vi "GE 5565 Dual Card.vi"() -> ()   [LabVIEW 2016]
uses:
  <vilib>/Utility/RT CPU Load.ctl
  <vilib>/Platform/TimedLoop/XDataNode/timing_clust.ctl
  <vilib>/Platform/TimedLoop/XDataNode/nitl_modes.ctl
  <vilib>/Platform/TimedLoop/XDataNode/wakeup.ctl
  <instrlib>/GE 5565 PIORC/Public/DMA Interrupt/GE5565 DMA Read Interrupt (U8) Cluster.vi
  <vilib>/Platform/TimedLoop/XDataNode/XDataNode.xnode
  <instrlib>/GE 5565 PIORC/GE 5565 PIORC.lvlib
  <vilib>/Platform/TimedLoop/XDataNode/XDNodeRunTimeDep.lvlib
  <vilib>/NI_Real-Time Target Support.lvlib
panel:
  out "w period 2":u32
  out "Times":cluster{u32, u32}
  out "CPU loads":T1[](array[typedef]) {"ISR (%)" format="%#.2f"; "Idle (%)" format="%#.2f"; "Background (%)" format="%#.2f"; "Normal (%)" format="%#.2f"; "Above Normal (%)" format="%#.2f"; "High (%)" format="%#.2g"; "Timed Structures (%)" format="%#.2g"; "Time Critical (%)" format="%#.2g"; "Total (%)" format="%#.2g"}
  in  "mode":enum16{"write", "read"}(ring)
  in  "size":i32=10000
  out "r element":dbl
  in  "r index":i32
  out "r period":u32
  in  "w element":dbl
  in  "w index":i32
  in  "stop":bool
  out "w period":u32
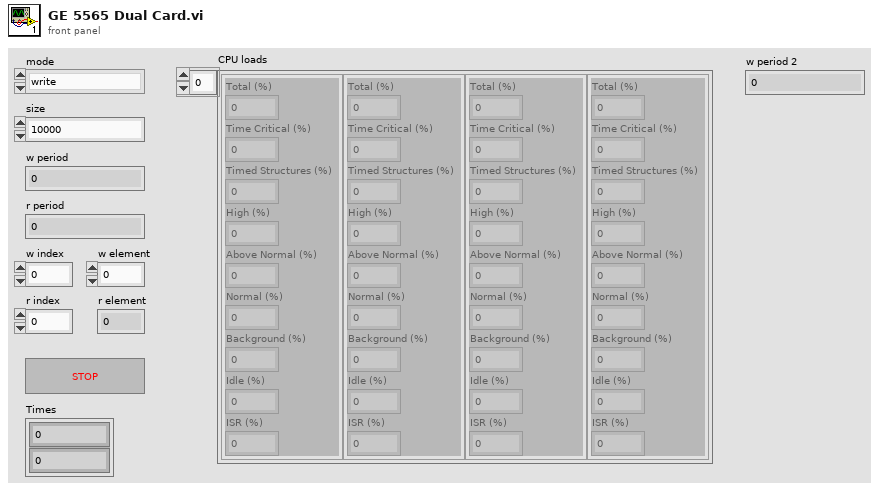
[diagram p1: front panel]
types:
  T1 = typedef "NI_Real-Time Target Support.lvlib/RT CPU Load.ctl" = cluster{"Total (%)":dbl, "Time Critical (%)":dbl, "Timed Structures (%)":dbl, "High (%)":dbl, "Above Normal (%)":dbl, "Normal (%)":dbl, "Background (%)":dbl, "Idle (%)":dbl, "ISR (%)":dbl}
  T2 = typedef "XDNodeRunTimeDep.lvlib/timing_clust.ctl" = cluster{"Expected End [f-1]":u64, "Actual End [f-1]":u64, "Finished Late? [f-1]":bool, "Expected End [i-1]":u64, "Actual End [i-1]":u64, "Finished Late? [i-1]":bool, "Expected Start [i]":u64, "Actual Start [i]":u64, "Expected Start [f]":u64, "Actual Start [f]":u64, "Source Name":string, "Structure Name":string, "Period":i64, "Deadline":i64, "Offset":i64, "Start":i64, "Priority":i32, "Timeout":i32, "Mode":T3, "Wakeup Reason":T4, "Error":errorcluster, "Source Type":string, "Secondary Source Type":string, "Global End Time":u64, "Global Start Time":u64, "Frame Duration":u64, "Iteration Duration":u64, "Assigned CPU":i32, "I/O Scan Engine Mode":u32}
  T3 = typedef "XDNodeRunTimeDep.lvlib/nitl_modes.ctl" = enum32{"No Change", "Process missed periods, maintain original phase", "Discard missed periods, maintain original phase", "Process missed periods, ignore original phase", "Discard missed periods, ignore original phase"}
  T4 = typedef "XDNodeRunTimeDep.lvlib/wakeup.ctl" = enum32{"Normal", "Aborted", "Asynchronous wakeup", "Timing source error", "Timed loop error", "Timeout"}
  T5 = cluster{"VMIC 5565 Resource":refnum<visa-resource-name>, "MEMACC Resource":refnum<visa-resource-name>, "byte count":u32, "mem offset":u32}
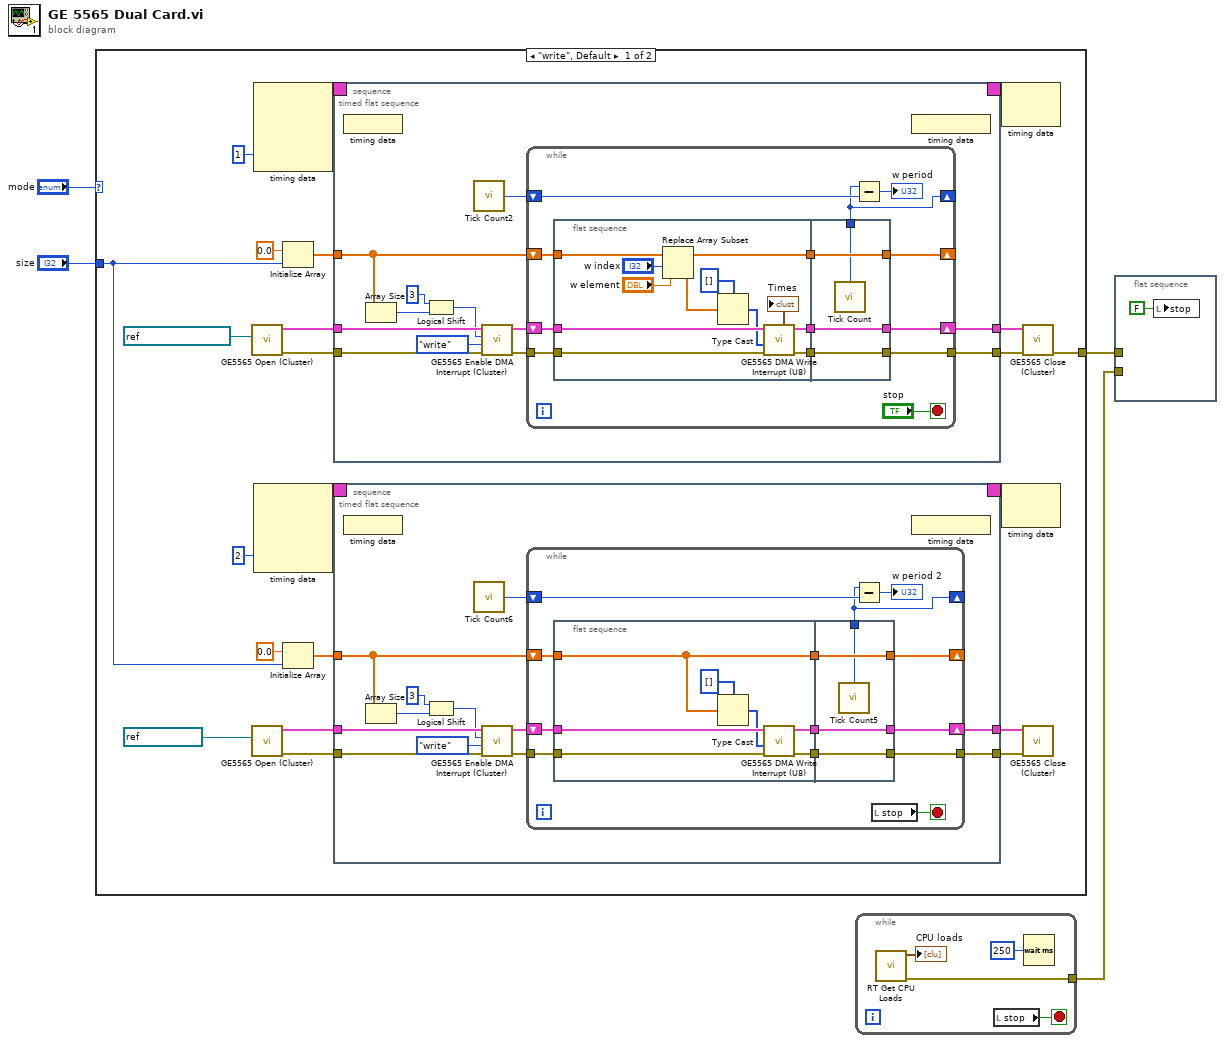
[diagram p0: block diagram]
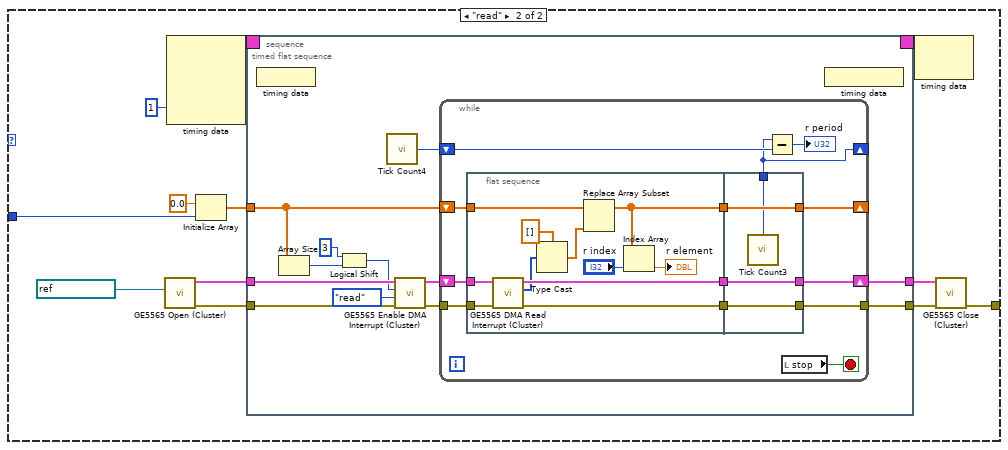
[diagram p2: hidden frame]
diagram:
  n1 = case shown="\"write\", Default" "mode" {
    tunnel: "size" -> [w15 w126]
    tunnel: [w16 w125] -> w2
    frame "write", Default {
      n2 = call <instrlib>:"GE5565 Open (Cluster).vi"("VISA resource name (empty)"=refnum<visa-resource-name> "PXI2::13::INSTR") -> ("error out"=w22:errorcluster, "VMIC-5565"=w23:T5)  [unwired: 5 in]
      n3 = call <instrlib>:"GE5565 Open (Cluster).vi"("VISA resource name (empty)"=refnum<visa-resource-name> "RefMem2") -> ("error out"=w7:errorcluster, "VMIC-5565"=w6:T5)  [unwired: 5 in]
      n4 = node-c288(1 ("Processor")) -> (w26:T2)  [unwired: 3 in]
      n5 = node-c288(2 ("Processor")) -> (w14:T2)  [unwired: 3 in]
      n6 = Initialize Array(0.0 ("element"), w15) -> (w18:dbl[])
      n7 = Initialize Array(0.0 ("element"), w15) -> (w11:dbl[])
      n8 = timed-sequence {
        timing: w26 -> [_]
        timing-out: [_] -> w25
        tunnel: w23 -> [w78]
        tunnel: w22 -> [w77]
        tunnel: [w76] -> w21
        tunnel: [w75] -> w20
        tunnel: w18 -> [w74]
        n9 = timed-flat-sequence {
          tunnel: w78 -> [w90]
          tunnel: w77 -> [w89]
          tunnel: [w87] -> w76
          tunnel: [w85] -> w75
          tunnel: w74 -> [w84]
          n10 = node-c288() -> ()  [unwired: 1 in]
          n11 = Array Size(array=w84) -> (size(s)=w83:i32)
          n12 = Logical Shift(y=i16 3, x=w83) -> (x << y=w81:i32)
          n13 = call "Tick Count2"() -> ("Tick Count(uSec)"=w79:u32)
          n14 = call <instrlib>:"GE5565 Enable DMA Interrupt (Cluster).vi"("error in (no error)"=w89, "operation (read)"=enum16{"read", "write"}."write", "transfer size (1024 bytes)"=w81, "VMIC reference in"=w90) -> ("error out"=w86:errorcluster, "VMIC reference out"=w88:T5)  [unwired: 2 in]
          n15 = while {
            shift-right: [w101] -> w87
            shift-left: w88 -> [w103]
            tunnel: w86 -> [w102]
            tunnel: [w100] -> w85
            shift-right: [w96] -> _
            shift-left: w84 -> [w99]
            shift-right: [w92] -> _
            shift-left: w79 -> [w95]
            stop <- "stop" stop-if-true
            n16 = flat-sequence {
              tunnel: w103 -> [w109]
              tunnel: w102 -> [w108]
              tunnel: w99 -> [w113]
              tunnel: [w107] -> w98
              tunnel: [w112] -> w97
              tunnel: [w106] -> w91
              tunnel: [w116] -> w96
              tunnel: [w117] -> w100
              tunnel: [w118] -> w101
              tunnel: w98 -> [w117]
              tunnel: w97 -> [w116]
              tunnel: [w115] -> w92
              tunnel: w91 -> [w118]
              frame #0 {
                n17 = Replace Array Subset(array=w113, new element="w element", index="w index") -> (w112:dbl[])
                n18 = Type Cast(type=u8[] [], x=w112) -> (*(type *) &x=w105:u8[])
                n19 = call "GE5565 DMA Write Interrupt (U8).vi"("error in (no error)"=w108, "buffer"=w105, "VMIC reference in"=w109) -> ("error out"=w107:errorcluster, "VMIC reference out"=w106:T5, "Times"=→"Times":cluster{u32, u32})  [unwired: 6 in]
              }
              frame #1 {
                n20 = call "Tick Count"() -> ("Tick Count(uSec)"=w115:u32)
              }
            }
            n21 = Subtract(x=w92, y=w95) -> (x-y=→"w period":u32)
          }
          n22 = node-c288() -> ()  [unwired: 1 out]
        }
      }
      n23 = timed-sequence {
        timing: w14 -> [_]
        timing-out: [_] -> w13
        tunnel: w6 -> [w31]
        tunnel: w7 -> [w30]
        tunnel: [w29] -> w8
        tunnel: [w28] -> w9
        tunnel: w11 -> [w27]
        n24 = timed-flat-sequence {
          tunnel: w31 -> [w43]
          tunnel: w30 -> [w42]
          tunnel: [w40] -> w29
          tunnel: [w38] -> w28
          tunnel: w27 -> [w37]
          n25 = node-c288() -> ()  [unwired: 1 in]
          n26 = Array Size(array=w37) -> (size(s)=w36:i32)
          n27 = Logical Shift(y=i16 3, x=w36) -> (x << y=w34:i32)
          n28 = call "Tick Count6"() -> ("Tick Count(uSec)"=w32:u32)
          n29 = call <instrlib>:"GE5565 Enable DMA Interrupt (Cluster).vi"("error in (no error)"=w42, "operation (read)"=enum16{"read", "write"}."write", "transfer size (1024 bytes)"=w34, "VMIC reference in"=w43) -> ("error out"=w39:errorcluster, "VMIC reference out"=w41:T5)  [unwired: 2 in]
          n30 = while {
            shift-right: [w54] -> w40
            shift-left: w41 -> [w56]
            tunnel: w39 -> [w55]
            tunnel: [w53] -> w38
            shift-right: [w49] -> _
            shift-left: w37 -> [w52]
            shift-right: [w46] -> _
            shift-left: w32 -> [w48]
            stop <- w44 stop-if-true
            n31 = flat-sequence {
              tunnel: w56 -> [w62]
              tunnel: w55 -> [w61]
              tunnel: w52 -> [w57]
              tunnel: [w60] -> w51
              tunnel: [w57] -> w50
              tunnel: [w59] -> w45
              tunnel: [w65] -> w49
              tunnel: [w66] -> w53
              tunnel: [w67] -> w54
              tunnel: w51 -> [w66]
              tunnel: w50 -> [w65]
              tunnel: [w64] -> w46
              tunnel: w45 -> [w67]
              frame #0 {
                n32 = Type Cast(type=u8[] [], x=w57) -> (*(type *) &x=w58:u8[])
                n33 = call "GE5565 DMA Write Interrupt (U8).vi"("error in (no error)"=w61, "buffer"=w58, "VMIC reference in"=w62) -> ("error out"=w60:errorcluster, "VMIC reference out"=w59:T5)  [unwired: 6 in, 1 out]
              }
              frame #1 {
                n34 = call "Tick Count5"() -> ("Tick Count(uSec)"=w64:u32)
              }
            }
            n35 = Subtract(x=w46, y=w48) -> (x-y=→"w period 2":u32)
            n36 = local read "stop"() -> (w44:bool)
          }
          n37 = node-c288() -> ()  [unwired: 1 out]
        }
      }
      n38 = node-c288(w25) -> ()  [unwired: 1 out]
      n39 = node-c288(w13) -> ()  [unwired: 1 out]
      n40 = call <instrlib>:"GE5565 Close (Cluster).vi"("error in (no error)"=w20, "VMIC reference in"=w21) -> ("error out"=w16:errorcluster)  [unwired: 5 in]
      n41 = call <instrlib>:"GE5565 Close (Cluster).vi"("error in (no error)"=w9, "VMIC reference in"=w8) -> ()  [unwired: 5 in, 1 out]
    }
    frame "read" {
      n42 = call <instrlib>:"GE5565 Open (Cluster).vi"("VISA resource name (empty)"=refnum<visa-resource-name> "RefMem2") -> ("error out"=w132:errorcluster, "VMIC-5565"=w133:T5)  [unwired: 5 in]
      n43 = node-c288(1 ("Processor")) -> (w136:T2)  [unwired: 3 in]
      n44 = Initialize Array(0.0 ("element"), w126) -> (w128:dbl[])
      n45 = timed-sequence {
        timing: w136 -> [_]
        timing-out: [_] -> w135
        tunnel: w133 -> [w141]
        tunnel: w132 -> [w140]
        tunnel: [w139] -> w131
        tunnel: [w138] -> w130
        tunnel: w128 -> [w137]
        n46 = timed-flat-sequence {
          tunnel: w141 -> [w153]
          tunnel: w140 -> [w152]
          tunnel: [w150] -> w139
          tunnel: [w148] -> w138
          tunnel: w137 -> [w147]
          n47 = node-c288() -> ()  [unwired: 1 in]
          n48 = Array Size(array=w147) -> (size(s)=w146:i32)
          n49 = Logical Shift(y=i16 3, x=w146) -> (x << y=w144:i32)
          n50 = call "Tick Count4"() -> ("Tick Count(uSec)"=w142:u32)
          n51 = call <instrlib>:"GE5565 Enable DMA Interrupt (Cluster).vi"("error in (no error)"=w152, "operation (read)"=enum16{"read", "write"}."read", "transfer size (1024 bytes)"=w144, "VMIC reference in"=w153) -> ("error out"=w149:errorcluster, "VMIC reference out"=w151:T5)  [unwired: 2 in]
          n52 = while {
            shift-right: [w164] -> w150
            shift-left: w151 -> [w166]
            tunnel: w149 -> [w165]
            tunnel: [w163] -> w148
            shift-right: [w158] -> _
            shift-left: w147 -> [w162]
            shift-right: [w155] -> _
            shift-left: w142 -> [w157]
            stop <- w154 stop-if-true
            n53 = flat-sequence {
              tunnel: w166 -> [w176]
              tunnel: w165 -> [w174]
              tunnel: w162 -> [w171]
              tunnel: [w173] -> w161
              tunnel: [w175] -> w160
              tunnel: [w167] -> w159
              tunnel: [w179] -> w158
              tunnel: [w180] -> w163
              tunnel: [w181] -> w164
              tunnel: w161 -> [w181]
              tunnel: w160 -> [w180]
              tunnel: w159 -> [w179]
              tunnel: [w178] -> w155
              frame #0 {
                n54 = call-poly <instrlib>:"GE5565 DMA Read Interrupt (Cluster).vi"("error in (no error)"=w174, "VMIC reference in"=w176) -> ("error out"=w175:errorcluster, "buffer"=w172:u8[], "VMIC reference out"=w173:T5)  [unwired: 7 in]
                n55 = Type Cast(type=dbl[] [], x=w172) -> (*(type *) &x=w170:dbl[])
                n56 = Replace Array Subset(array=w171, new element=w170) -> (w167:dbl[])  [unwired: 1 in]
                n57 = Index Array(array=w167, index="r index") -> (element=→"r element":dbl)
              }
              frame #1 {
                n58 = call "Tick Count3"() -> ("Tick Count(uSec)"=w178:u32)
              }
            }
            n59 = Subtract(x=w155, y=w157) -> (x-y=→"r period":u32)
            n60 = local read "stop"() -> (w154:bool)
          }
          n61 = node-c288() -> ()  [unwired: 1 out]
        }
      }
      n62 = node-c288(w135) -> ()  [unwired: 1 out]
      n63 = call <instrlib>:"GE5565 Close (Cluster).vi"("error in (no error)"=w130, "VMIC reference in"=w131) -> ("error out"=w125:errorcluster)  [unwired: 5 in]
    }
  }
  n64 = while {
    tunnel: [w188] -> w1
    stop <- w191 stop-if-true
    n65 = call <vilib>:"RT Get CPU Loads.vi"() -> ("error out"=w188:errorcluster, "CPU loads"=→"CPU loads":T1[])  [unwired: 10 in]
    n66 = local read "stop"() -> (w191:bool)
    n67 = Wait (ms)(milliseconds to wait=u32 250) -> ()  [unwired: 1 out]
  }
  n68 = flat-sequence {
    tunnel: w2 -> [_]
    tunnel: w1 -> [_]
    frame #0 {
      n69 = local write "stop"(FALSE ("stop")) -> ()
    }
  }
